vi "Write Kitchen.vi"(8 "error in (no error)":errorcluster, 10 "Kitcher Message Enqueuer":refnum<class "Message Enqueuer.lvclass">, 11 "COOKING in":refnum<class "COOKING.lvclass">) -> (0 "error out":errorcluster, 3 "COOKING out":refnum<class "COOKING.lvclass">)   [LabVIEW 2024, in "Chef States.lvlib" / "COOKING.lvclass"]
uses:
  COOKING.lvclass
  COOKING.lvclass/COOKING.ctl
  <vilib>/ActorFramework/Message Enqueuer/Message Enqueuer.lvclass
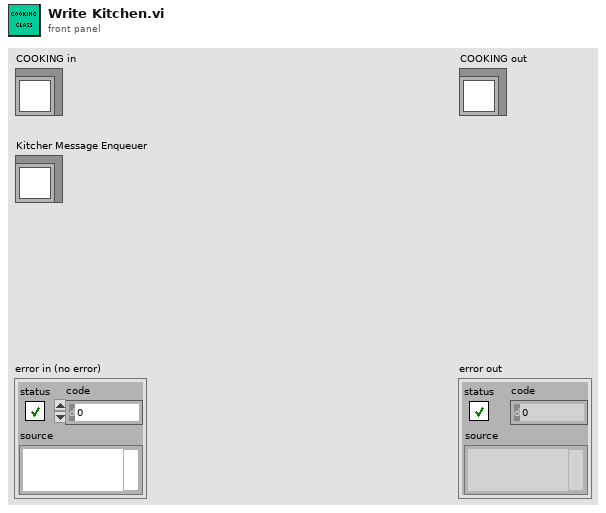
[diagram p1: front panel]
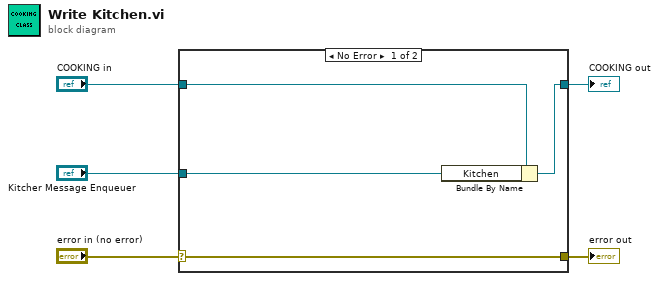
[diagram p0: block diagram]
diagram:
  n1 = case shown="No Error" "error in (no error)" {
    selector: "error in (no error)" -> [w9 w10]
    tunnel: [w9 w10] -> w4
    tunnel: [w7 w11] -> w2
    tunnel: "COOKING in" -> [w8 w11]
    tunnel: "Kitcher Message Enqueuer" -> [w6 _]
    frame No Error {
      n2 = Bundle By Name(cluster=w8, "Kitchen"=w6) -> (w7:refnum<class "COOKING.lvclass">)
    }
    frame Error {
    }
  }
  "error out" <- w4
  "COOKING out" <- w2
